vi "IsHorizontal.vi"(9 "Slide in":refnum<class "Slide.lvclass">) -> (3 "Slide out":refnum<class "Slide.lvclass">, 4 "horizontal":bool)   [LabVIEW 2014, in "Slide.lvclass"]
uses:
  Slide.lvclass
  Control/Control.lvclass/Control.ctl
  Control/Control.lvclass
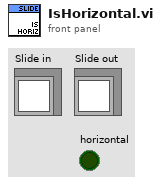
[diagram p1: front panel]
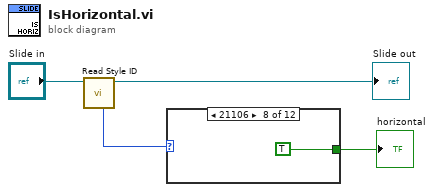
[diagram p0: block diagram]
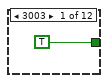
[diagram p2: hidden frame]
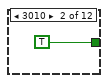
[diagram p3: hidden frame]
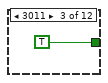
[diagram p4: hidden frame]
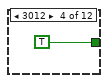
[diagram p5: hidden frame]
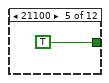
[diagram p6: hidden frame]
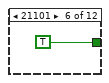
[diagram p7: hidden frame]
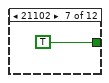
[diagram p8: hidden frame]
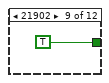
[diagram p9: hidden frame]
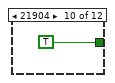
[diagram p10: hidden frame]
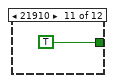
[diagram p11: hidden frame]
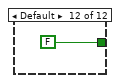
[diagram p12: hidden frame]
diagram:
  n1 = call "Read Style ID.vi"("Control in"="Slide in") -> ("Control out"=→"Slide out":refnum<class "Slide.lvclass">, "Style ID"=w3:u32)  [unwired: 7 in]
  n2 = case shown="21106" w3 {
    tunnel: [TRUE TRUE TRUE TRUE TRUE TRUE TRUE TRUE TRUE TRUE TRUE FALSE] -> w2
    frame 3003 {
    }
    frame 3010 {
    }
    frame 3011 {
    }
    frame 3012 {
    }
    frame 21100 {
    }
    frame 21101 {
    }
    frame 21102 {
    }
    frame 21106 {
    }
    frame 21902 {
    }
    frame 21904 {
    }
    frame 21910 {
    }
    frame Default {
    }
  }
  "horizontal" <- w2
